vi "Initialize.vi"(6 "SerialSetting":T1={"Baud Rate"=115200, "Data Bits"=8, "Parity"=0, "Stop Bits"=10} {"Stop Bits" items=["1.0"=10, "1.5"=15, "2.0"=20]; "Parity" items=["None", "Odd", "Even", "Mark", "Space"]}, 8 "error in (no error)":errorcluster, 9 "Reset (True)":bool=TRUE, 10 "ID Query (True)":bool=TRUE, 11 "VISA resource name":refnum<visa-resource-name>) -> (0 "error out":errorcluster, 2 "ID information":T2, 3 "VISA resource name out":refnum<visa-resource-name>)   [LabVIEW 2020, in "GPP.lvlib"]
uses:
  GPP.lvlib
  Function/VISA_COMMON.ctl
panel:
  # "(c) 2005-2008 National Instruments.  ALL RIGHTS RESERVED."
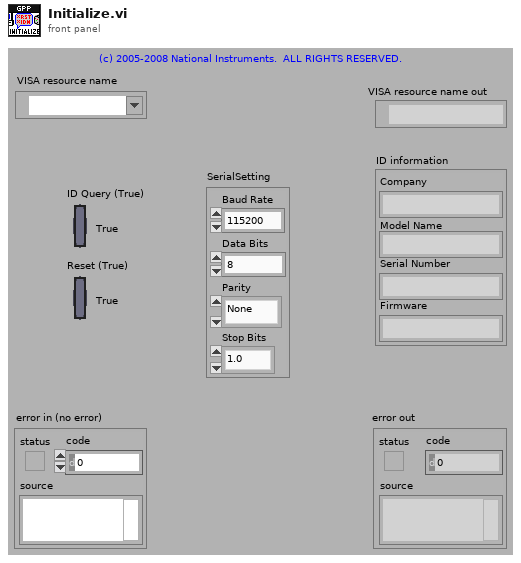
[diagram p1: front panel]
types:
  T1 = cluster{"Baud Rate":u32, "Data Bits":u16, "Parity":u16, "Stop Bits":u16}
  T2 = cluster{"Company":string, "Model Name":string, "Serial Number":string, "Firmware":string}
  T3 = typedef "GPP.lvlib/VISA_COMMON.ctl" = enum16{"Initial", "Write CMD", "Read Result", "Read History", "Close"}
  T4 = cluster{"[0]":string, "[1]":string, "[2]":string, "[3]":string}
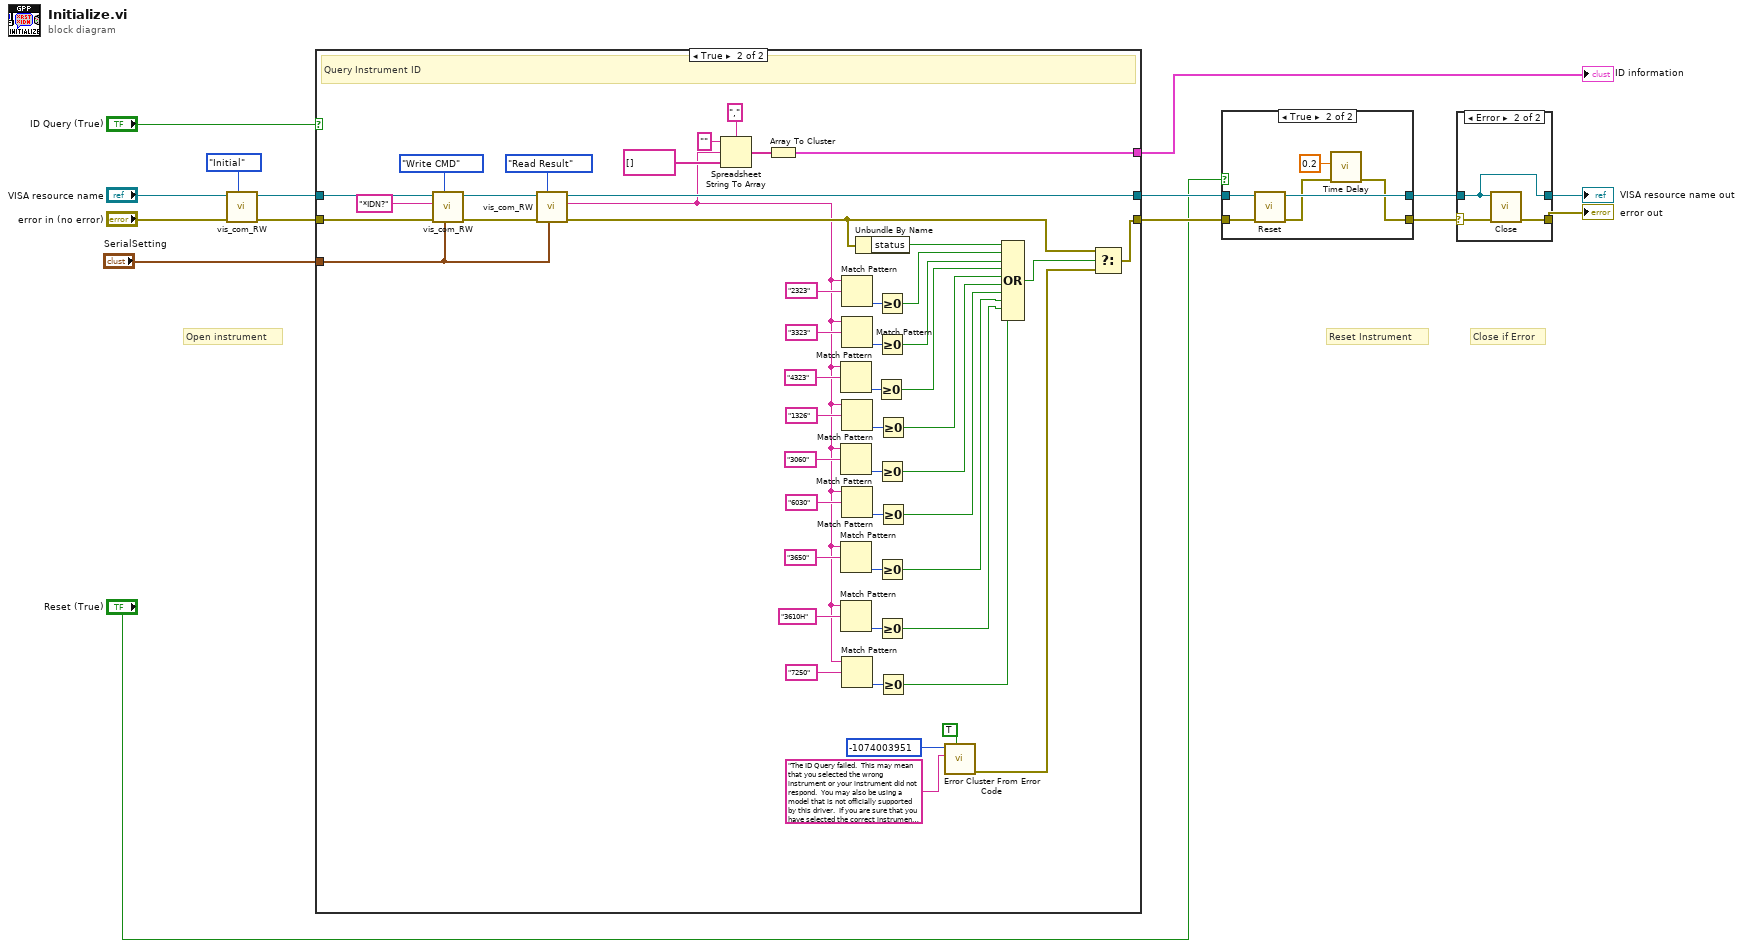
[diagram p0: block diagram]
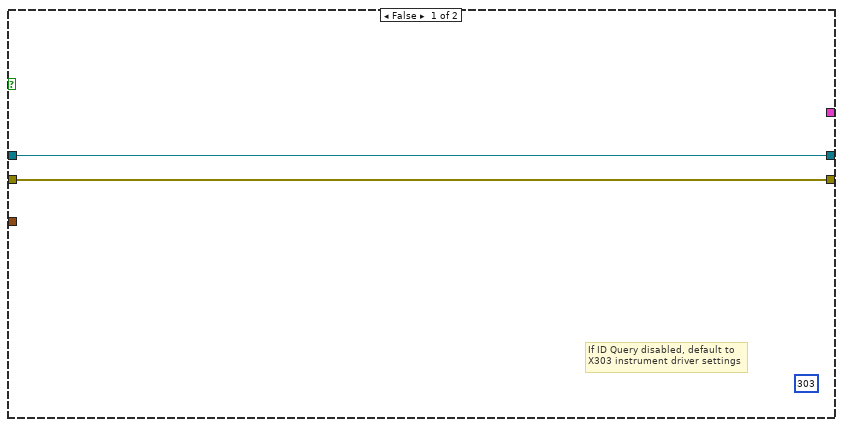
[diagram p3: hidden frame]
diagram:
  # "Close if Error"
  # "Reset Instrument"
  # "Open instrument"
  n1 = call "vis_com_RW.vi"("Funciton"=VISA_COMMON."Initial", "error in (no error)"="error in (no error)", "VISA resource in"="VISA resource name") -> ("error out"=w8:errorcluster, "VISA resource out"=w9:refnum<visa-resource-name>)  [unwired: 6 in, 1 out]
  n2 = case shown="True" "ID Query (True)" {
    tunnel: [w16 w67] -> w4
    tunnel: [w17 w42] -> w6
    tunnel: w9 -> [w17 w45]
    tunnel: w8 -> [w16 w46]
    tunnel: [_ w35] -> w7
    tunnel: "SerialSetting" -> [_ w34]
    frame False {
      (unwired) 303
      # "If ID Query disabled, default to X303 instrument driver settings"
    }
    frame True {
      # "Query Instrument ID"
      n3 = call "vis_com_RW.vi"("SerialSetting"=w34, "Funciton"=VISA_COMMON."Write CMD", "error in (no error)"=w46, "CMD String"="*IDN?" ("ID Query"), "VISA resource in"=w45) -> ("error out"=w40:errorcluster, "VISA resource out"=w43:refnum<visa-resource-name>)  [unwired: 4 in, 1 out]
      n4 = call "vis_com_RW.vi"("SerialSetting"=w34, "Funciton"=VISA_COMMON."Read Result", "error in (no error)"=w40, "VISA resource in"=w43) -> ("error out"=w41:errorcluster, "Result"=w18:string, "VISA resource out"=w42:refnum<visa-resource-name>)  [unwired: 5 in]
      n5 = Spreadsheet String To Array(delimiter (Tab)=",", format string="", spreadsheet string=w18, array type (2D Dbl)=string[] []) -> (array=w37:string[])
      n6 = Array To Cluster(array=w37) -> (cluster=w35:T4)
      n7 = Match Pattern(string=w18, regular expression="4323") -> (offset past match=w54:i32)  [unwired: 4 out]
      n8 = Match Pattern(string=w18, regular expression="3060") -> (offset past match=w32:i32)  [unwired: 4 out]
      n9 = Match Pattern(string=w18, regular expression="3650") -> (offset past match=w26:i32)  [unwired: 4 out]
      n10 = Match Pattern(string=w18, regular expression="3610H") -> (offset past match=w25:i32)  [unwired: 4 out]
      n11 = Match Pattern(string=w18, regular expression="2323") -> (offset past match=w61:i32)  [unwired: 4 out]
      n12 = Match Pattern(string=w18, regular expression="3323") -> (offset past match=w59:i32)  [unwired: 4 out]
      n13 = Match Pattern(string=w18, regular expression="1326") -> (offset past match=w51:i32)  [unwired: 4 out]
      n14 = Match Pattern(string=w18, regular expression="6030") -> (offset past match=w31:i32)  [unwired: 4 out]
      n15 = Match Pattern(string=w18, regular expression="7250") -> (offset past match=w22:i32)  [unwired: 4 out]
      n16 = Unbundle By Name(w41) -> ("status"=w60:bool)
      n17 = Greater Or Equal To 0?(x=w54) -> (x >= 0?=w52:bool)
      n18 = Greater Or Equal To 0?(x=w61) -> (x >= 0?=w57:bool)
      n19 = Greater Or Equal To 0?(x=w59) -> (x >= 0?=w53:bool)
      n20 = Greater Or Equal To 0?(x=w32) -> (x >= 0?=w29:bool)
      n21 = Greater Or Equal To 0?(x=w26) -> (x >= 0?=w21:bool)
      n22 = Greater Or Equal To 0?(x=w25) -> (x >= 0?=w20:bool)
      n23 = Greater Or Equal To 0?(x=w51) -> (x >= 0?=w50:bool)
      n24 = Greater Or Equal To 0?(x=w31) -> (x >= 0?=w28:bool)
      n25 = Greater Or Equal To 0?(x=w22) -> (x >= 0?=w19:bool)
      n26 = call <vilib>:"Error Cluster From Error Code.vi"("show call chain? (False)"=TRUE, "error message (\"\")"="The ID Query failed.  This may mean that you selected the wrong instrument or your instrument did not respond.  You may also be using a model that is not officially supported by this driver.  If you are sure that you have selected the correct instrument and it is responding, try disabling the ID Query." ("Source (VI Name)"), "error code (0)"=-1074003951 ("Code")) -> ("error out"=w65:errorcluster)  [unwired: 1 in, 5 out]
      n27 = Compound Arithmetic op=OR(w60, w57, w53, w52, w50, w29, w28, w21, w20, w19) -> (w56:bool)
      n28 = Select(t=w41, s=w56, f=w65) -> (s? t:f=w67:errorcluster)
    }
  }
  "ID information" <- w7
  n29 = case shown="True" "Reset (True)" {
    tunnel: w6 -> [w69 w75]
    tunnel: [w69 w74] -> w5
    tunnel: w4 -> [w68 w73]
    tunnel: [w68 w71] -> w3
    frame False {
    }
    frame True {
      n30 = call "Reset.vi"("error in (no error)"=w73, "VISA resource name"=w75) -> ("error out"=w72:errorcluster, "VISA resource name out"=w74:refnum<visa-resource-name>)  [unwired: 8 in]
      n31 = call "Time Delay"("error in (no error)"=w72, "Delay Time (s)"=0.2) -> ("error out"=w71:errorcluster)  [unwired: 9 in]
    }
  }
  n32 = case shown="Error" w3 {
    selector: w3 -> [w76 w79]
    tunnel: w5 -> [w77 w78]
    tunnel: [w77 w78] -> w15
    tunnel: [w76 w80] -> w13
    frame No Error {
    }
    frame Error {
      n33 = call "Close.vi"("error in (no error)"=w79, "VISA resource name"=w78) -> ("error out"=w80:errorcluster)  [unwired: 9 in]
    }
  }
  "VISA resource name out" <- w15
  "error out" <- w13
